vi "Get Datatype group.vi"(8 "error in (no error)":errorcluster, 10 "name":string, 11 "Channel group in":refnum<class "Channel group.lvclass">) -> (0 "error out":errorcluster, 1 "Datatype group":refnum<class "Datatype group.lvclass">, 2 "found":bool, 3 "Channel group out":refnum<class "Channel group.lvclass">)   [LabVIEW 2016, in "FPGA RM Shared API.lvlib" / "Channel group.lvclass"]
uses:
  Channel group.lvclass
  Datatype Group/Datatype group.lvclass
  Channel group.lvclass/Channel group.ctl
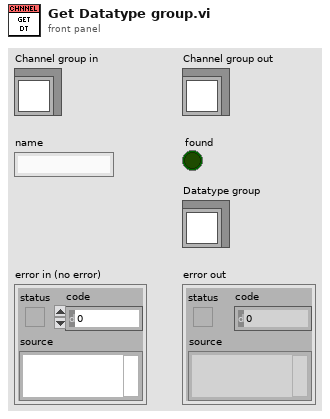
[diagram p1: front panel]
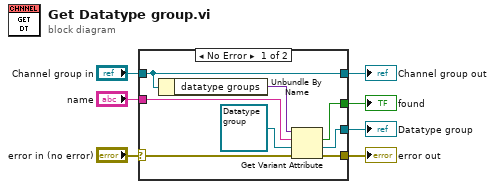
[diagram p0: block diagram]
diagram:
  n1 = case shown="No Error" "error in (no error)" {
    selector: "error in (no error)" -> [w12 w17]
    tunnel: [w11 w17] -> w6
    tunnel: [w15 w16] -> w4
    tunnel: "Channel group in" -> [w15 w16]
    tunnel: "name" -> [w13 _]
    tunnel: [w9 _] -> w2
    tunnel: [w8 _] -> w1
    frame No Error {
      n2 = Unbundle By Name(w15) -> ("datatype groups"=w14:variant)
      n3 = Get Variant Attribute(Variant=w14, name=w13, default value (empty Variant)=refnum<class "Datatype group.lvclass"> refnum ("FPGA RM Shared API.lvlib:Datatype group.lvclass"), error in=w12) -> (found=w8:bool, value=w9:refnum<class "Datatype group.lvclass">, error out=w11:errorcluster)  [unwired: 1 out]
    }
    frame Error {
    }
  }
  "error out" <- w6
  "Channel group out" <- w4
  "Datatype group" <- w2
  "found" <- w1
